vi "sample3(BasicRW ALL).vi"() -> ()   [LabVIEW 2020]
panel:
  out "Name/ModelNo":u16(ring) format="%04x" items=["XL320"=350, "H54-200-S500-R"=54024, "H54-100-S500-R"=53768, "H42-20-S300-R"=51200, "M54-60-S250-R"=46352, "M54-40-S250-R"=46096, "M42-10-S260-R"=43288, "L54-50-S290-R"=38176, "L54-50-S500-R"=38152, "L54-30-S400-R"=37928, "L54-30-S500-R"=37896, "L42-10-S300-R"=35072, "XM430-W350-R"=1020, "XM430-W210-R"=1030, "XH430-W350-R"=1000, "XH430-W210-R"=1010]
  in  "UPDATE":bool
  out "ACK":bool
  out "HW Error":T1
  in  "TorqueEnable":bool
  in  "OffsetTime":u32=500
  out "err":errorcluster caption="エラー出力" {"code" format="%04x"}
  in  "ID":u8=1 max=253
  in  "Baudrate":u32=57600 min=9600 max=3000000 step=100
  in  "COM":refnum<visa-resource-name> caption="COMポート"
  in  "STOP":bool
  in  "POSITION":i32(knob) min=-131594 max=131594
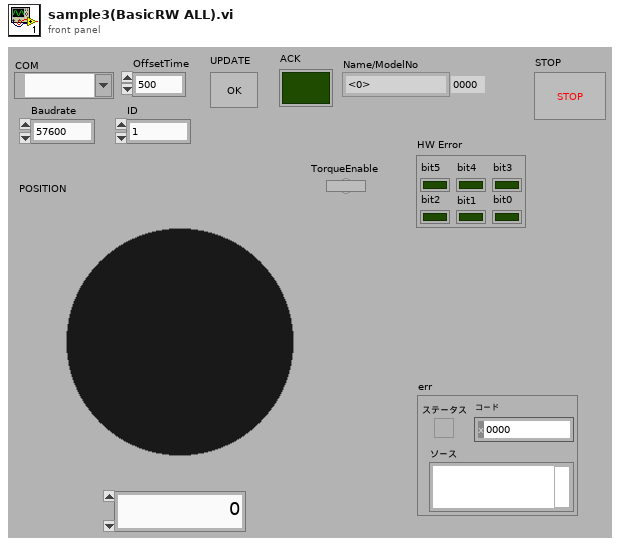
[diagram p1: front panel]
types:
  T1 = cluster{"bit0":bool, "bit1":bool, "bit2":bool, "bit3":bool, "bit4":bool, "bit5":bool}
  T2 = cluster{"Input Voltage":bool, "Motor hall sensor":bool, "Over Heating":bool, "Motor encorder":bool, "Electronical shock":bool, "Overload":bool}
  T3 = cluster{"tena":u16, "gpos":u16, "ppos":u16, "hwer":u16, "long":bool}
  T4 = cluster{"Boolean array[0]":bool, "Boolean array[1]":bool, "Boolean array[2]":bool, "Boolean array[3]":bool, "Boolean array[4]":bool, "Boolean array[5]":bool}
  T5 = cluster{"Name/ModelNo":u16, "Type":u8, "MaxPosition":i32, "MinPosition":i32, "ScaleFactor":dbl}
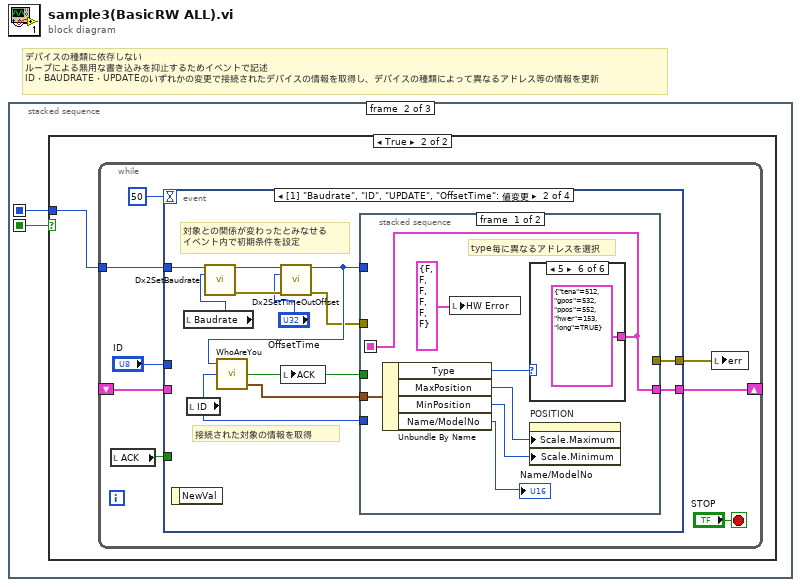
[diagram p0: block diagram]
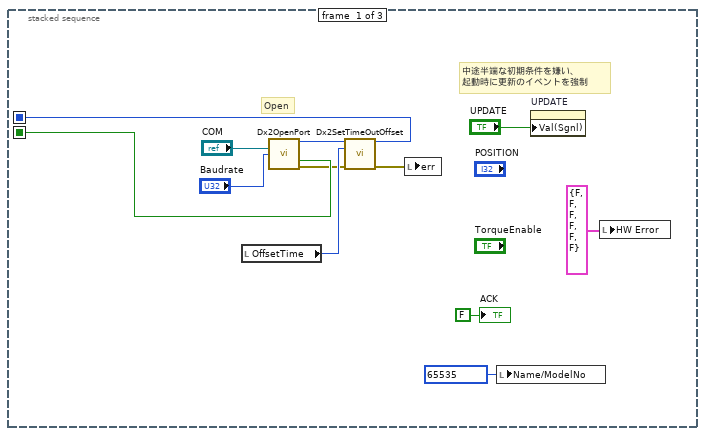
[diagram p2: hidden frame]
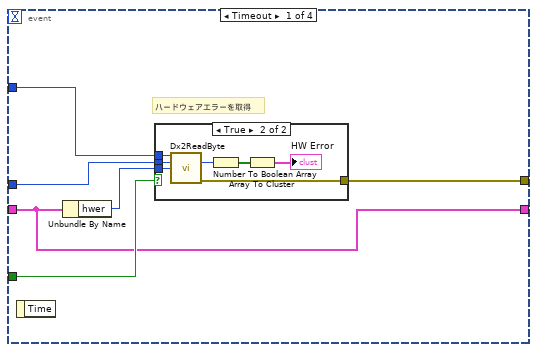
[diagram p4: hidden frame]
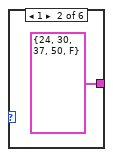
[diagram p7: hidden frame]
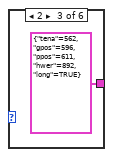
[diagram p8: hidden frame]
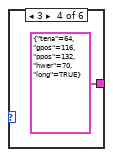
[diagram p9: hidden frame]
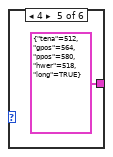
[diagram p10: hidden frame]
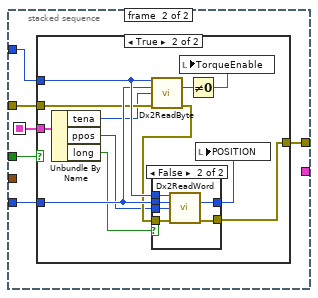
[diagram p11: hidden frame]
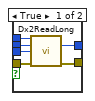
[diagram p13: hidden frame]
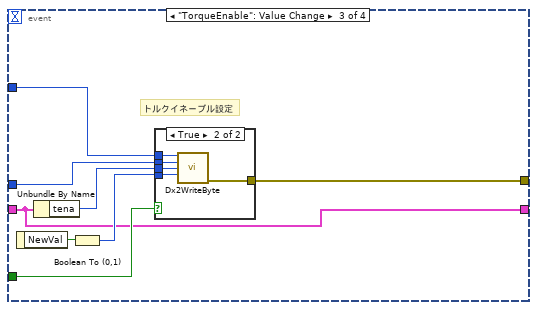
[diagram p14: hidden frame]
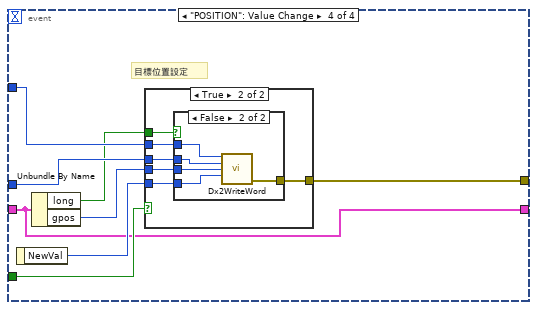
[diagram p16: hidden frame]
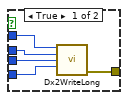
[diagram p18: hidden frame]
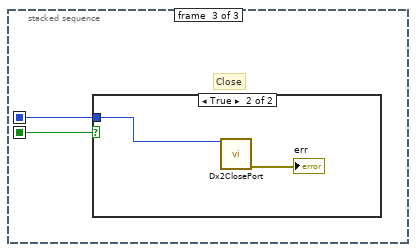
[diagram p19: hidden frame]
diagram:
  # "デバイスの種類に依存しない\nループによる無用な書き込みを抑止するためイベントで記述\nID・BAUDRATE・UPDATEのいずれかの変更で接続されたデバイスの情報を取得し、デバイスの種類によって異なるアドレス等の情報を更新"
  n1 = stacked-sequence {
    seq-local: [w1 _ _] -> [_ w14 w130]
    seq-local: [w10 _ _] -> [_ w13 w129]
    frame #0 {
      w6 = u16 65535 items=["XL320"=350, "H54-200-S500-R"=54024, "H54-100-S500-R"=53768, "H42-20-S300-R"=51200, "M54-60-S250-R"=46352, "M54-40-S250-R"=46096, "M42-10-S260-R"=43288, "L54-50-S290-R"=38176, "L54-50-S500-R"=38152, "L54-30-S400-R"=37928, "L54-30-S500-R"=37896, "L42-10-S300-R"=35072, "XM430-W350-R"=1020, "XM430-W210-R"=1030, "XH430-W350-R"=1000, "XH430-W210-R"=1010] ("Name/ModelNo")
      # "Open"
      # "中途半端な初期条件を嫌い、\n起動時に更新のイベントを強制"
      n2 = local read "OffsetTime"() -> (w4:u32)
      n3 = call "Dx2OpenPort.vi"("port"="COM", "baudrate"="Baudrate") -> ("dvid"=w5:u32, "成功"=w10:bool, "エラー出力"=w3:errorcluster)  [unwired: 11 in]
      n4 = call "Dx2SetTimeOutOffset.vi"("dvid in"=w5, "OffsetTime"=w4, "エラー入力"=w3) -> ("dvid out"=w1:u32, "エラー出力"=w2:errorcluster)  [unwired: 11 in]
      n5 = local write "err"(w2) -> ()
      n6 = local write "Name/ModelNo"(w6) -> ()
      n7 = property on="UPDATE" class="Bool (指定)"("Val(Sgnl)"="UPDATE") -> ()  [unwired: 2 in, 2 out]
      n8 = local write "HW Error"(T2 {"Input Voltage"=FALSE, "Motor hall sensor"=FALSE, "Over Heating"=FALSE, "Motor encorder"=FALSE, "Electronical shock"=FALSE, "Overload"=FALSE} ("HW Error")) -> ()
      "ACK" <- FALSE ("ACK")
    }
    frame #1 {
      n9 = case shown="TRUE" w13 {
        tunnel: w14 -> [_ w15]
        frame False {
        }
        frame True {
          n10 = while {
            tunnel: w15 -> [w19]
            shift-right: [w18] -> _
            shift-left: _ -> [w17]
            stop <- "STOP" stop-if-true
            n11 = local read "ACK"() -> (w16:bool)
            n12 = event shown="[1] \"Baudrate\", \"ID\", \"UPDATE\", \"OffsetTime\": 値変更" {
              selector: _ -> [_ _ _ _]
              dyn-events: _ -> [_ _ _ _]
              timeout: 50 -> [_ _ _ _]
              tunnel: "ID" -> [w29 _ w99 w111]
              tunnel: [w26 w44 w98 w112] -> w20
              tunnel: w19 -> [w27 w48 w95 w109]
              tunnel: [w24 w43 w92 w105] -> w18
              tunnel: w17 -> [w24 _ w92 w105]
              tunnel: w16 -> [w25 _ w93 w106]
              event Timeout {
                # "ハードウェアエラーを取得"
                n13 = event-data() -> ()  [unwired: 1 in, 1 out]
                n14 = Unbundle By Name(w24) -> ("hwer"=w28:u16)
                n15 = case shown="TRUE" w25 {
                  tunnel: w29 -> [_ w36]
                  tunnel: w28 -> [_ w32]
                  tunnel: w27 -> [_ w31]
                  tunnel: [_ w30] -> w26
                  frame False {
                  }
                  frame True {
                    n16 = call "Dx2ReadByte.vi"("dvid in"=w31, "id"=w36, "address"=w32) -> ("data out"=w34:u8, "エラー出力"=w30:errorcluster)  [unwired: 9 in, 2 out]
                    n17 = Number To Boolean Array(number=w34) -> (Boolean array=w35:bool[])
                    n18 = Array To Cluster(array=w35) -> (cluster=→"HW Error":T4)
                  }
                }
              }
              event "Baudrate", "ID", "UPDATE", "OffsetTime": Value Change {
                # "接続された対象の情報を取得"
                # "対象との関係が変わったとみなせる\nイベント内で初期条件を設定"
                n19 = event-data() -> ()  [unwired: 1 in, 1 out]
                n20 = local read "Baudrate"() -> (w47:u32)
                n21 = local read "ID"() -> (w42:u8)
                n22 = call "Dx2SetBaudrate.vi"("dvid in"=w48, "Baudrate"=w47) -> ("dvid out"=w41:u32, "エラー出力"=w39:errorcluster)  [unwired: 11 in, 1 out]
                n23 = call "Dx2SetTimeOutOffset.vi"("dvid in"=w41, "OffsetTime"="OffsetTime", "エラー入力"=w39) -> ("dvid out"=w40:u32, "エラー出力"=w38:errorcluster)  [unwired: 11 in]
                n24 = call "WhoAreYou.vi"("Target ID"=w42, "dvid in"=w40) -> ("TargetInfo"=w46:T5, "matched"=w45:bool)  [unwired: 1 in, 1 out]
                n25 = local write "ACK"(w45) -> ()
                n26 = stacked-sequence {
                  seq-local: [w51 _] -> [_ w61]
                  tunnel: w46 -> [w52 _]
                  tunnel: w45 -> [_ w66]
                  tunnel: w38 -> [_ w65]
                  tunnel: [_ w64] -> w44
                  tunnel: w40 -> [_ w63]
                  tunnel: w42 -> [_ w62]
                  tunnel: [w51 _] -> w43
                  frame #0 {
                    # "type毎に異なるアドレスを選択"
                    n27 = Unbundle By Name(w52) -> ("Type"=w53:u8, "MaxPosition"=w54:i32, "MinPosition"=w55:i32, "Name/ModelNo"=→"Name/ModelNo":u16)
                    n28 = local write "HW Error"(T2 {"Input Voltage"=FALSE, "Motor hall sensor"=FALSE, "Over Heating"=FALSE, "Motor encorder"=FALSE, "Electronical shock"=FALSE, "Overload"=FALSE} ("HW Error")) -> ()
                    n29 = case shown="5" w53 {
                      tunnel: [_ T3 {"tena"=24, "gpos"=30, "ppos"=37, "hwer"=50, "long"=FALSE} T3 {"tena"=562, "gpos"=596, "ppos"=611, "hwer"=892, "long"=TRUE} T3 {"tena"=64, "gpos"=116, "ppos"=132, "hwer"=70, "long"=TRUE} T3 {"tena"=512, "gpos"=564, "ppos"=580, "hwer"=518, "long"=TRUE} T3 {"tena"=512, "gpos"=532, "ppos"=552, "hwer"=153, "long"=TRUE}] -> w51
                      frame 0, Default {
                      }
                      frame 1 {
                      }
                      frame 2 {
                      }
                      frame 3 {
                      }
                      frame 4 {
                      }
                      frame 5 {
                      }
                    }
                    n30 = property on="POSITION" class="Knob (指定)"("Scale.Maximum"=w54, "Scale.Minimum"=w55) -> ()  [unwired: 2 in, 2 out]
                  }
                  frame #1 {
                    n31 = case shown="TRUE" w66 {
                      tunnel: w63 -> [_ w79]
                      tunnel: w62 -> [_ w78]
                      tunnel: w65 -> [w67 w77]
                      tunnel: [w67 w75] -> w64
                      tunnel: w61 -> [_ w68]
                      frame False {
                      }
                      frame True {
                        n32 = Unbundle By Name(w68) -> ("tena"=w69:u16, "ppos"=w70:u16, "long"=w71:bool)
                        n33 = call "Dx2ReadByte.vi"("dvid in"=w79, "id"=w78, "address"=w69, "エラー入力"=w77) -> ("data out"=w74:u8, "エラー出力"=w76:errorcluster)  [unwired: 8 in, 2 out]
                        n34 = case shown="FALSE" w71 {
                          tunnel: w79 -> [w85 w91]
                          tunnel: w78 -> [w84 w90]
                          tunnel: w70 -> [w83 w89]
                          tunnel: w76 -> [w82 w88]
                          tunnel: [w81 w87] -> w75
                          tunnel: [w80 w86] -> w72
                          frame True {
                            n35 = call "Dx2ReadLong.vi"("dvid in"=w85, "id"=w84, "address"=w83, "エラー入力"=w82) -> ("data out"=w80:u32, "エラー出力"=w81:errorcluster)  [unwired: 8 in, 2 out]
                          }
                          frame False {
                            n36 = call "Dx2ReadWord.vi"("dvid in"=w91, "id"=w90, "address"=w89, "エラー入力"=w88) -> ("data out"=w86:u16, "エラー出力"=w87:errorcluster)  [unwired: 8 in, 2 out]
                          }
                        }
                        n37 = Not Equal To 0?(x=w74) -> (x != 0?=w73:bool)
                        n38 = local write "TorqueEnable"(w73) -> ()
                        n39 = local write "POSITION"(w72) -> ()
                      }
                    }
                  }
                }
              }
              event "TorqueEnable": Value Change {
                # "トルクイネーブル設定"
                n40 = event-data() -> ("NewVal"=w97:bool)  [unwired: 1 in]
                n41 = Unbundle By Name(w92) -> ("tena"=w94:u16)
                n42 = Boolean To (0,1)(Boolean=w97) -> (0, 1=w96:i16)
                n43 = case shown="TRUE" w93 {
                  tunnel: w99 -> [_ w104]
                  tunnel: [_ w103] -> w98
                  tunnel: w96 -> [_ w102]
                  tunnel: w95 -> [_ w101]
                  tunnel: w94 -> [_ w100]
                  frame False {
                  }
                  frame True {
                    n44 = call "Dx2WriteByte.vi"("dvid in"=w101, "id"=w104, "address"=w100, "data in"=w102) -> ("エラー出力"=w103:errorcluster)  [unwired: 9 in, 2 out]
                  }
                }
              }
              event "POSITION": Value Change {
                # "目標位置設定"
                n45 = event-data() -> ("NewVal"=w110:i32)  [unwired: 1 in]
                n46 = Unbundle By Name(w105) -> ("long"=w108:bool, "gpos"=w107:u16)
                n47 = case shown="TRUE" w106 {
                  tunnel: [_ w118] -> w112
                  tunnel: w111 -> [_ w117]
                  tunnel: w110 -> [_ w116]
                  tunnel: w109 -> [_ w115]
                  tunnel: w108 -> [_ w114]
                  tunnel: w107 -> [_ w113]
                  frame False {
                  }
                  frame True {
                    n48 = case shown="FALSE" w114 {
                      tunnel: [w123 w128] -> w118
                      tunnel: w115 -> [w122 w127]
                      tunnel: w117 -> [w121 w126]
                      tunnel: w116 -> [w120 w125]
                      tunnel: w113 -> [w119 w124]
                      frame True {
                        n49 = call "Dx2WriteLong.vi"("dvid in"=w122, "id"=w121, "address"=w119, "data in"=w120) -> ("エラー出力"=w123:errorcluster)  [unwired: 9 in, 2 out]
                      }
                      frame False {
                        n50 = call "Dx2WriteWord.vi"("dvid in"=w127, "id"=w126, "address"=w124, "data in"=w125) -> ("エラー出力"=w128:errorcluster)  [unwired: 9 in, 2 out]
                      }
                    }
                  }
                }
              }
            }
            n51 = local write "err"(w20) -> ()
          }
        }
      }
    }
    frame #2 {
      # "Close"
      n52 = case shown="TRUE" w129 {
        tunnel: w130 -> [_ w132]
        frame False {
        }
        frame True {
          n53 = call "Dx2ClosePort.vi"("dvid"=w132) -> ("エラー出力"=→"err":errorcluster)  [unwired: 13 in, 1 out]
        }
      }
    }
  }
